vi "Control - Industrial Control.vi"() -> ()   [LabVIEW 2013, in "PID Control Workspace Object.lvlib"]
doc: "Sample numeric display item."
uses:
  Control Workspace Object Support.llb/PID Control Workspace Object.lvlib
  NationalInstruments.VeriStand.SystemStorage
  NationalInstruments.VeriStand.ClientAPI
  Control Workspace Object Support.llb/Constants.vi
  Control Workspace Object Support.llb/Control Addon Shared.lvlib
  Control Workspace Object Support.llb/NI_VS Workspace ExecutionAPI.lvlib
panel:
  in  "Manual State":bool
  in  "Manual Control":bool
  in  "Setpoint":dbl
  in  "NIVS.System Definition Root":refnum<k24>
  in  "NIVS.Gateway IP Address":string
  in  "Hold":bool
  in  "Autoscale Y":bool=TRUE
  in  "Autoscale X":bool=TRUE
  out "Chart":waveform(dbl)[](graph)
  out "Control Name":string
  in  "Item.Data":T1
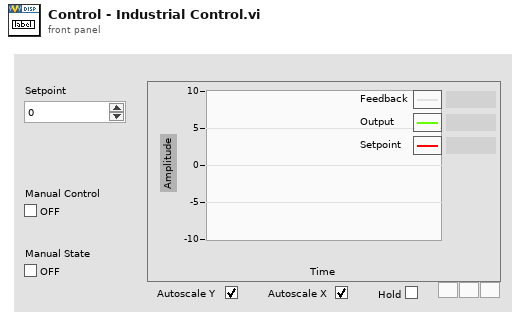
[diagram p1: front panel]
types:
  T1 = cluster{"Template VI":string, "Position X":i32, "Position Y":i32, "Custom":string, "Show Title Bar":bool, "ID":i32, "Always On Top":bool, "Allow Resize":bool, "Allow Minimize":bool, "Allow Close":bool, "Size to Screen":bool, "Screen.ID":i32, "State":enum16{"Normal", "New"}, "Title":string, "Window Bounds":cluster{"[0]":i16, "[1]":i16, "[2]":i16, "[3]":i16}, "Channel Ref":u64, "Unit":string, "Default Units?":bool, "Flash Limit?":bool, "Color 1":u32, "Color 2":u32, "Color 3":u32, "Color 4":u32, "Bck Color":u32, "Fore Color":u32, "Limit 1":dbl, "Limit 2":dbl, "Limit 3":dbl, "Limit 4":dbl, "Limit Mode 1":i32, "Limit Mode 2":i32, "Limit Mode 3":i32, "Limit Mode 4":i32, "Scale Precision":i32, "Scale Min":dbl, "Scale Max":dbl, "Format":i32, "Precision":i32, "Background Type":i32, "IDs":i32[], "Units":string[], "Labels":string[], "Scale Factor":dbl, "Scale Offset":dbl, "YScale Index":u32[], "XScale":cluster{"Format":u8, "Precision":u8, "Fit":u8, "Label":string, "Use Default Label":bool, "Label Visible":bool, "Min":dbl, "Max":dbl}, "YScales":cluster{"Format":u8, "Precision":u8, "Fit":u8, "Label":string, "Use Default Label":bool, "Label Visible":bool, "Min":dbl, "Max":dbl}[], "Plots":cluster{"Bar Style":u8, "Fill To":i16, "Fill/PtColor":u32, "Line Style":u8, "Line Width":u8, "Color":u32, "Interp":u8, "Point Style":u8}[], "Update Period":dbl, "History Length":dbl, "My.Ref":refnum<vi>, "Is Control?":bool, "Channel Paths":string[], "Custom Data":variant}
  T2 = enum8{"Idle", "Start Acq", "Run", "Stop Acq", "Exit"}
  T3 = cluster{"Action":enum8{"Idle", "Start Acq", "Run", "Stop Acq", "Exit"}, "Channels":string[]}
  T4 = cluster{"Initialized Waveform":waveform(dbl)[], "VS UDP Session":refnum<k24>, "Channel IDs":i32[], "Packet IDs":i32[], "Max Packet Size":i32, "UDP Ref":refnum<k16>}
  T5 = cluster{"Cached":cluster{"Path":string}, "Found?":bool, "UDP Channels":string[], "Connected?":bool, "Previous Values":dbl[], "Slow Channels":string[]}
  T6 = cluster{"Operation":enum16{"SetCustomData", "DeleteItem"}, "Data":variant}
  T7 = cluster{"CustDatRef":refnum<user-event>, "EvtRef":refnum<k27>}
  T8 = cluster{"Event Registration Refnum":refnum<event-registration>, "SystemChangeEventRef":refnum<event-registration>}
  T9 = cluster{"ID":i32, "t0":dbl, "dt":dbl, "Channel IDs":i32[], "Channel Data":dbl[][], "Sample Offset":u64}
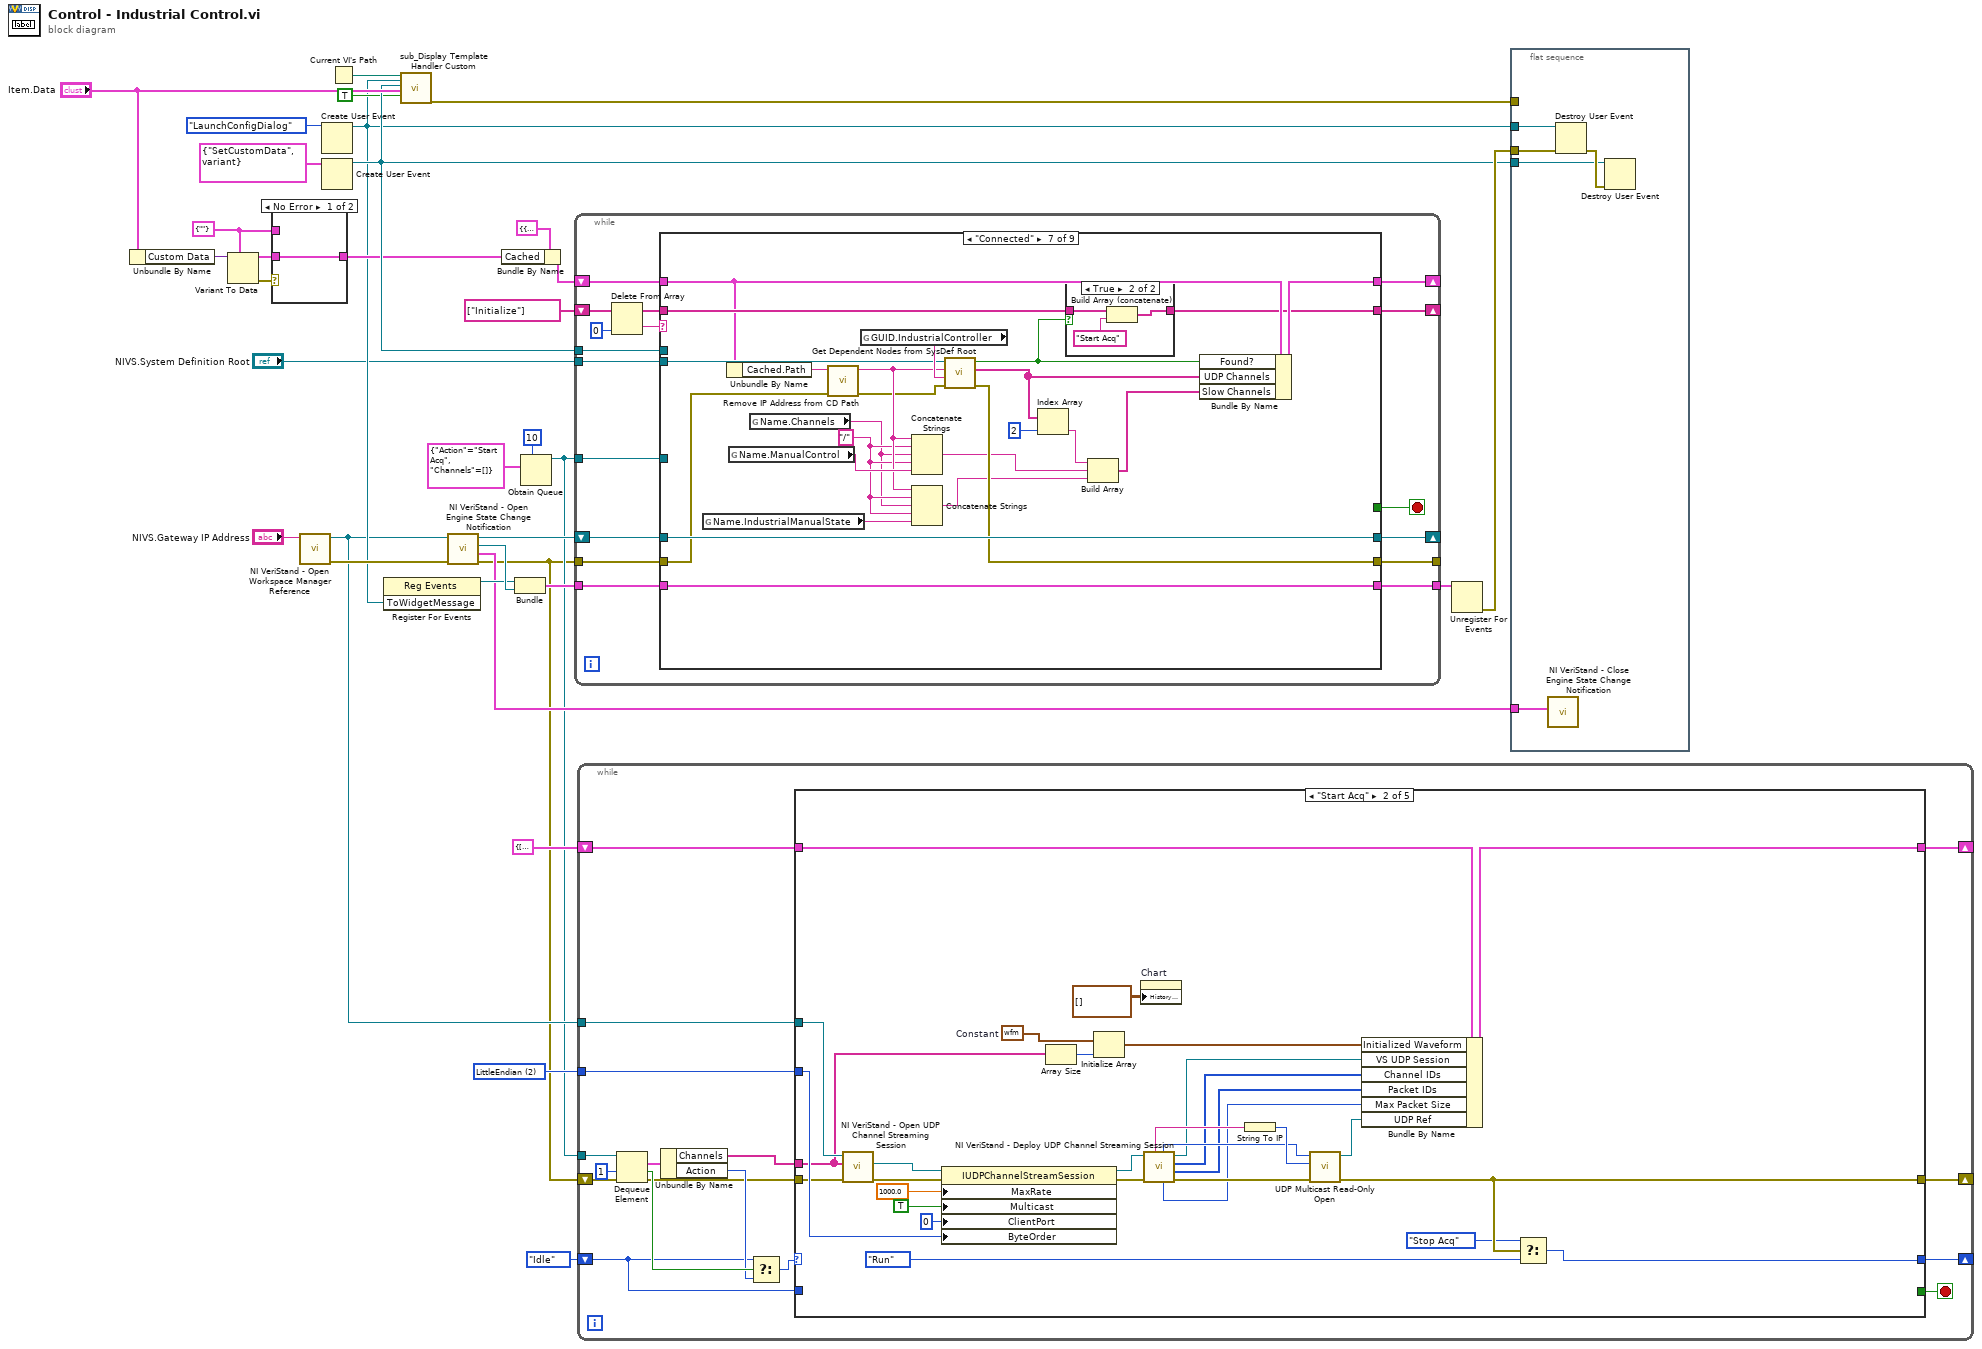
[diagram p0: block diagram]
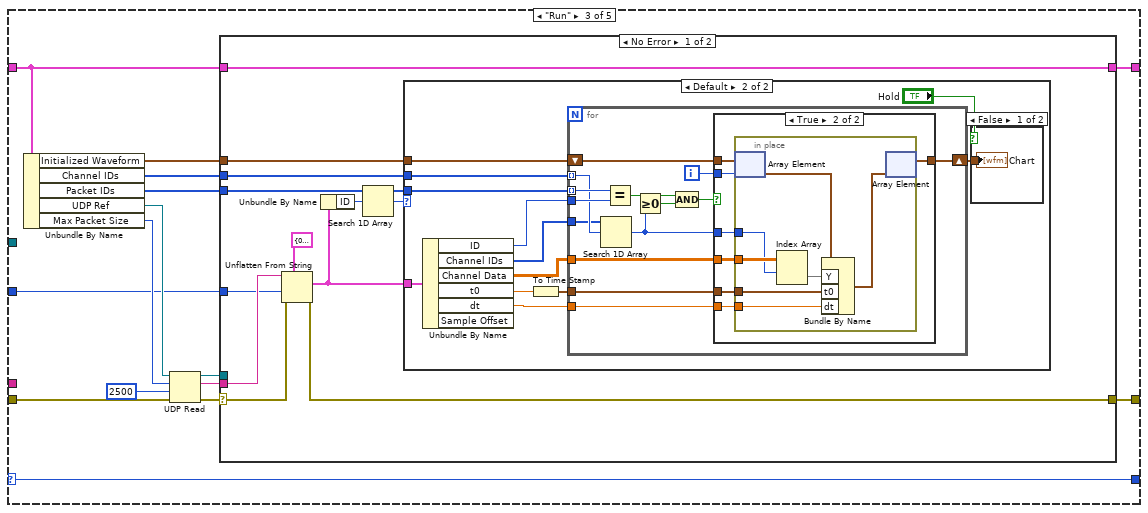
[diagram p3: hidden frame]
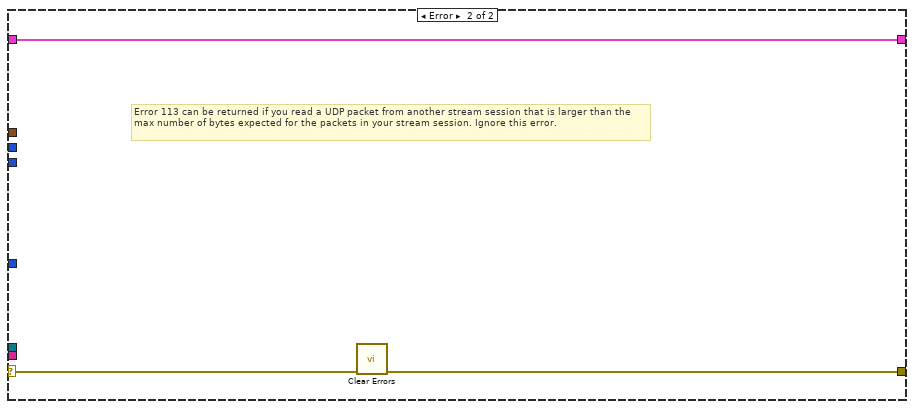
[diagram p7: hidden frame]
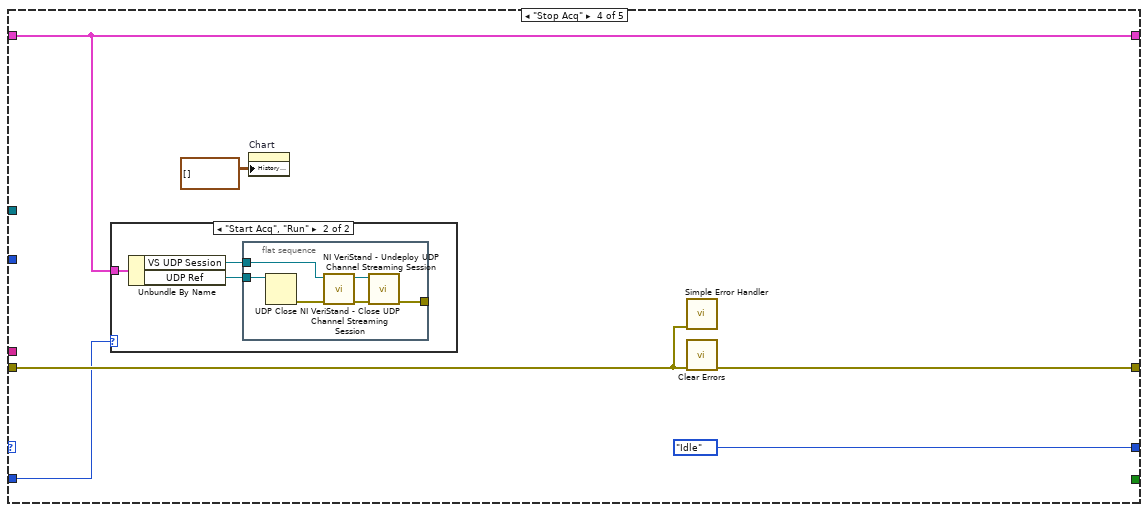
[diagram p8: hidden frame]
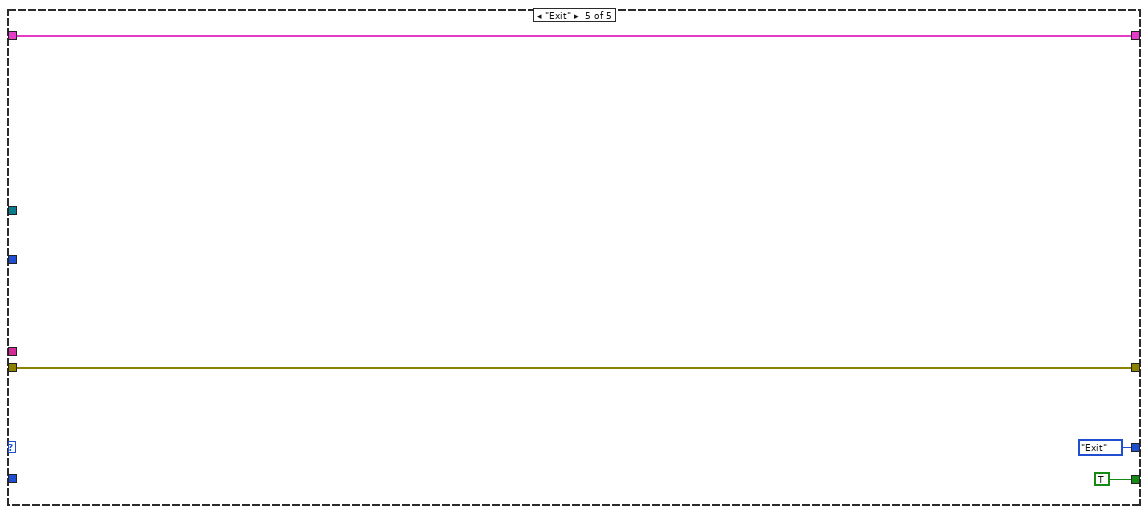
[diagram p10: hidden frame]
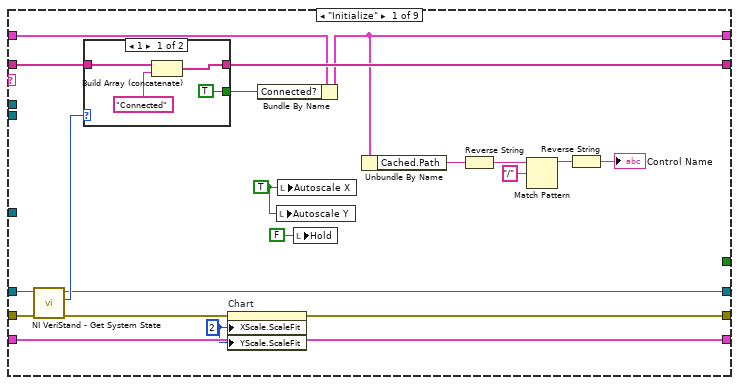
[diagram p12: hidden frame]
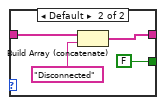
[diagram p13: hidden frame]
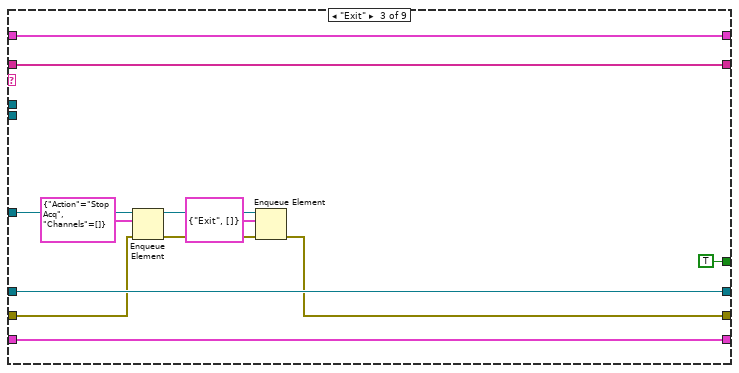
[diagram p15: hidden frame]
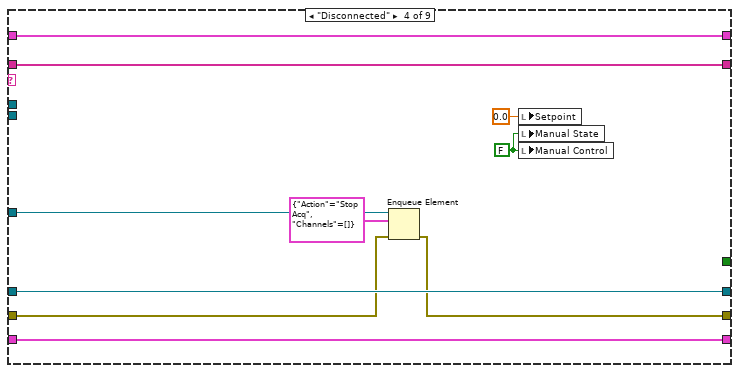
[diagram p16: hidden frame]
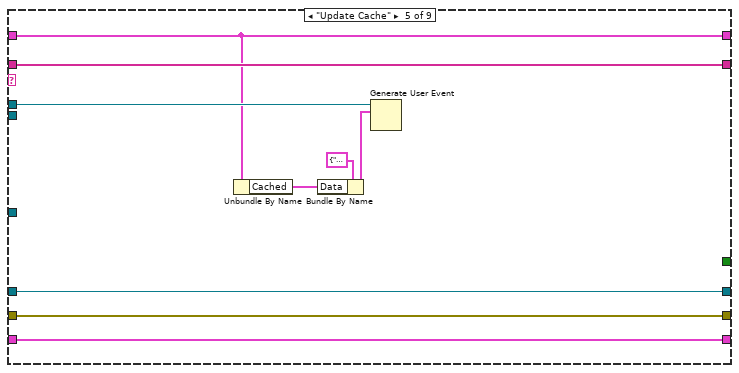
[diagram p17: hidden frame]
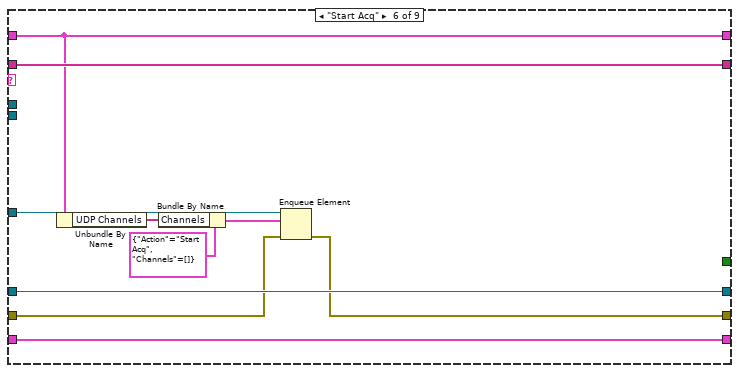
[diagram p18: hidden frame]
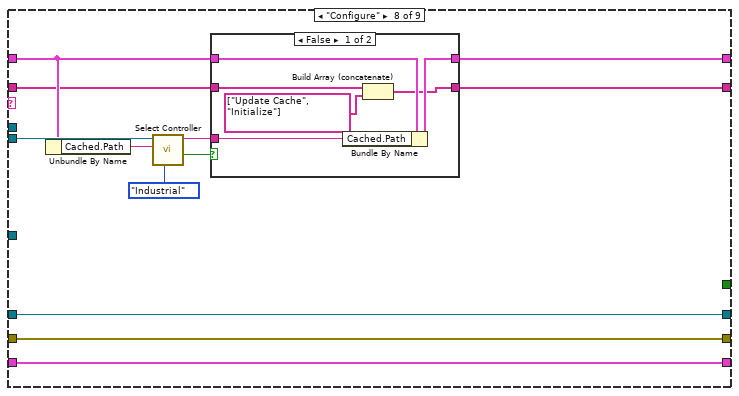
[diagram p20: hidden frame]
diagram:
  w6 = 2 items=["BigEndian", "NativeHostOrder", "LittleEndian"] ("Byte Order")
  w14 = cluster{"Path":string} {"Path"=""}
  n1 = Unbundle By Name("Item.Data") -> ("Custom Data"=w18:variant)
  n2 = Variant To Data(type=w14, Variant=w18) -> (data=w15:cluster{"Path":string}, error out=w16:errorcluster)  [unwired: 1 in]
  n3 = case shown="No Error" w16 {
    tunnel: w15 -> [w35 _]
    tunnel: [w35 w36] -> w11
    tunnel: w14 -> [_ w36]
    frame No Error {
    }
    frame Error {
    }
  }
  n4 = call "NI VeriStand - Open Workspace Manager Reference.vi"("Gateway IP Address (\"\": localhost)"="NIVS.Gateway IP Address") -> ("error out"=w25:errorcluster, "WorkspaceManager"=w8:refnum<k24>)  [unwired: 9 in]
  n5 = Create User Event(user event datatype=enum16{"Stop", "LaunchConfigDialog"}."LaunchConfigDialog" ("ToWidgetMessage")) -> (user event=w10:refnum<user-event>)  [unwired: 1 in, 1 out]
  n6 = Create User Event(user event datatype=T6 {"Operation"=enum."SetCustomData", "Data"=variant} ("Data")) -> (user event=w28:refnum<user-event>)  [unwired: 1 in, 1 out]
  n7 = Current VI's Path() -> (path=w30:path)
  n8 = register-events(w10) -> (reference out=w23:refnum<event-registration>)  [unwired: 2 in, 1 out]
  n9 = call "sub_Display Template Handler Custom.vi"("Parent.Path"=w30, "ToWidgetEvent"=w10, "ToWorkspace"=w28, "Item.Data"="Item.Data", "Resizable"=TRUE) -> ("error out"=w34:errorcluster)  [unwired: 14 in]
  n10 = call "NI VeriStand - Open Engine State Change Notification.vi"("error in (no error)"=w25, "WorkspaceManager in"=w8) -> ("error out"=w1:errorcluster, "SystemStateRefs"=w21:T7, "SystemChangeEventRef"=w24:refnum<event-registration>, "WorkspaceManager out"=w19:refnum<k24>)  [unwired: 6 in]
  n11 = Bundle By Name(cluster=T5 {"Cached"={"Path"=""}, "Found?"=FALSE, "UDP Channels"=[], "Connected?"=FALSE, "Previous Values"=[0.0, 0.0, 0.0], "Slow Channels"=[]}, "Cached"=w11) -> (w12:T5)
  n12 = Bundle("Event Registration Refnum"=w23, "SystemChangeEventRef"=w24) -> (w22:T8)  [unwired: 1 in]
  n13 = Obtain Queue(max queue size (-1, unlimited)=10, element data type=T3 {"Action"=enum."Start Acq", "Channels"=[]}) -> (queue out=w3:refnum<queue>)  [unwired: 3 in, 2 out]
  n14 = while {
    tunnel: w22 -> [w53]
    tunnel: w28 -> [w51]
    shift-right: [w45] -> _
    shift-left: string[] ["Initialize"] -> [w49]
    shift-right: [w43] -> _
    shift-left: w19 -> [w42]
    tunnel: w1 -> [w47]
    tunnel: [w44] -> w17
    tunnel: [w40] -> _
    shift-right: [w39] -> _
    shift-left: w12 -> [w41]
    tunnel: "NIVS.System Definition Root" -> [w38]
    tunnel: w3 -> [w37]
    stop <- w52 stop-if-true
    n15 = Delete From Array(array=w49, index=0) -> (deleted portion=w48:string, array with subset deleted=w46:string[])  [unwired: 1 in]
    n16 = case shown="\"Connected\"" w48 {
      tunnel: w53 -> [w67 w85 w97 w107 w116 w126 w150 w167 w186]
      tunnel: [_ _ TRUE _ _ _ _ _ _] -> w52
      tunnel: [w69 w86 w98 w108 w117 w127 w133 w157 w183] -> w45
      tunnel: w51 -> [_ _ _ _ w113 _ _ _ _]
      tunnel: w47 -> [w72 w83 w89 w103 w114 w119 w137 w165 w179]
      tunnel: w46 -> [w70 w86 w98 w108 w117 w127 w151 w156 w182]
      tunnel: [w67 w85 w97 w107 w116 w126 w150 w167 w184] -> w44
      tunnel: [w68 w84 w96 w106 w115 w125 w149 w166 w180] -> w43
      tunnel: w42 -> [w71 w84 w96 w106 w115 w125 w149 w166 w181]
      tunnel: w41 -> [w61 w82 w95 w105 w110 w124 w145 w161 w176]
      tunnel: [w55 w83 w88 w102 w114 w118 w148 w165 w178] -> w40
      tunnel: [w60 w82 w95 w105 w110 w124 w144 w160 w177] -> w39
      tunnel: w38 -> [_ _ _ _ _ _ w146 w163 _]
      tunnel: w37 -> [_ _ w94 w104 _ w123 _ _ _]
      frame "Initialize" {
        w57 = u8 2 ("X Scale.Scale Fit")
        w58 = TRUE ("Autoscale X")
        n17 = call "NI VeriStand - Get System State.vi"("error in (no error)"=w72, "WorkspaceManager in"=w71) -> ("error out"=w56:errorcluster, "System State"=w73:u8, "WorkspaceManager  out"=w68:refnum<k24>)  [unwired: 5 in, 2 out]
        n18 = case shown="1" w73 {
          tunnel: w70 -> [w77 w81]
          tunnel: [w76 w80] -> w69
          tunnel: [TRUE FALSE] -> w59
          frame 1 {
            n19 = Build Array (concatenate)(w77, "Connected") -> (w76:string[])
          }
          frame Default {
            n20 = Build Array (concatenate)(w81, "Disconnected") -> (w80:string[])
          }
        }
        n21 = property on="Chart" class="WFChart (strict)"(error in=w56, "XScale.ScaleFit"=w57, "YScale.ScaleFit"=w57) -> (error out=w55:errorcluster)  [unwired: 1 in, 1 out]
        n22 = Bundle By Name(cluster=w61, "Connected?"=w59) -> (w60:T5)
        n23 = local write "Autoscale Y"(w58) -> ()
        n24 = local write "Autoscale X"(w58) -> ()
        n25 = local write "Hold"(FALSE ("Hold")) -> ()
        n26 = Unbundle By Name(w60) -> ("Cached.Path"=w63:string)
        n27 = Reverse String(1:w63) -> (0:w66:string)
        n28 = Match Pattern(string=w66, regular expression="/") -> (before substring=w62:string)  [unwired: 1 in, 3 out]
        n29 = Reverse String(1:w62) -> (0:→"Control Name":string)
      }
      frame Default {
      }
      frame "Exit" {
        n30 = Enqueue Element(queue=w94, element=T3 {"Action"=enum."Stop Acq", "Channels"=[]}, error in (no error)=w89) -> (queue out=w92:refnum<queue>, error out=w90:errorcluster)  [unwired: 1 in, 1 out]
        n31 = Enqueue Element(queue=w92, element=T3 {"Action"=enum."Exit", "Channels"=[]}, error in (no error)=w90) -> (error out=w88:errorcluster)  [unwired: 1 in, 2 out]
      }
      frame "Disconnected" {
        w99 = FALSE ("Manual Control")
        n32 = Enqueue Element(queue=w104, element=T3 {"Action"=enum."Stop Acq", "Channels"=[]}, error in (no error)=w103) -> (error out=w102:errorcluster)  [unwired: 1 in, 2 out]
        n33 = local write "Setpoint"(0.0 ("Setpoint")) -> ()
        n34 = local write "Manual State"(w99) -> ()
        n35 = local write "Manual Control"(w99) -> ()
      }
      frame "Update Cache" {
        n36 = Unbundle By Name(w110) -> ("Cached"=w109:cluster{"Path":string})
        n37 = Bundle By Name(cluster=T6 {"Operation"=enum."SetCustomData", "Data"=variant} ("event data"), "Data"=w109) -> (w111:T6)
        n38 = Generate User Event(user event=w113, event data cluster=w111) -> ()  [unwired: 2 in, 2 out]
      }
      frame "Start Acq" {
        n39 = Unbundle By Name(w124) -> ("UDP Channels"=w121:string[])
        n40 = Bundle By Name(cluster=T3 {"Action"=enum."Start Acq", "Channels"=[]}, "Channels"=w121) -> (w120:T3)
        n41 = Enqueue Element(queue=w123, element=w120, error in (no error)=w119) -> (error out=w118:errorcluster)  [unwired: 1 in, 2 out]
      }
      frame "Connected" {
        w130 = "/" ("string")
        n42 = global read "Constants.vi" "Name.IndustrialManualState"() -> (w140:string)
        n43 = Unbundle By Name(w145) -> ("Cached.Path"=w143:string)
        n44 = global read "Constants.vi" "Name.ManualControl"() -> (w142:string)
        n45 = global read "Constants.vi" "Name.Channels"() -> (w129:string)
        n46 = call "Remove IP Address from CD Path.vi"("error in (no error)"=w137, "CD Path"=w143) -> ("error out"=w136:errorcluster, "Path"=w141:string)  [unwired: 8 in]
        n47 = global read "Constants.vi" "GUID.IndustrialController"() -> (w147:string)
        n48 = Concatenate Strings(w141, w130, w129, w130, w142) -> (w139:string)
        n49 = Concatenate Strings(w141, w130, w129, w130, w140) -> (w138:string)
        n50 = call "Get Dependent Nodes from SysDef Root.vi"("error in (no error)"=w136, "GUID"=w147, "Path"=w141, "SysDef Ref"=w146) -> ("error out"=w148:errorcluster, "Channels"=w132:string[], "Found"=w128:bool)  [unwired: 5 in]
        n51 = Index Array(array=w132, index=2) -> (element=w134:string)
        n52 = case shown="True" w128 {
          tunnel: w151 -> [w152 w155]
          tunnel: [w152 w154] -> w133
          frame False {
          }
          frame True {
            n53 = Build Array (concatenate)(w155, "Start Acq") -> (w154:string[])
          }
        }
        n54 = Build Array(w134, w139, w138) -> (w131:string[])
        n55 = Bundle By Name(cluster=w145, "Found?"=w128, "UDP Channels"=w132, "Slow Channels"=w131) -> (w144:T5)
      }
      frame "Configure" {
        n56 = Unbundle By Name(w161) -> ("Cached.Path"=w162:string)
        n57 = call "Select Controller.vi"("Type"=enum16{"PID", "Industrial"}."Industrial", "CD Path"=w162, "NIVS.System Definition Root"=w163) -> ("Cancelled?"=w159:bool, "Custom Device Path Out"=w158:string)  [unwired: 6 in, 1 out]
        n58 = case shown="False" w159 {
          tunnel: w161 -> [w173 w174]
          tunnel: [w172 w174] -> w160
          tunnel: w158 -> [w171 _]
          tunnel: [w169 w175] -> w157
          tunnel: w156 -> [w170 w175]
          frame False {
            n59 = Bundle By Name(cluster=w173, "Cached.Path"=w171) -> (w172:T5)
            n60 = Build Array (concatenate)(w170, string[] ["Update Cache", "Initialize"]) -> (w169:string[])
          }
          frame True {
          }
        }
      }
      frame "" {
        n61 = event shown="[2] \"Setpoint\", \"Manual Control\", \"Manual State\": Value Change" {
          selector: w186 -> [_ _ _ _ _]
          dyn-events: [_ _ _ _ _] -> w184
          timeout: 100 -> [_ _ _ _ _]
          tunnel: [w205 w227 w245 w274 w294] -> w183
          tunnel: w182 -> [w205 w227 w245 w275 w293]
          tunnel: w181 -> [w202 w226 w238 w278 w295]
          tunnel: [w201 w226 w237 w277 w295] -> w180
          tunnel: w179 -> [w204 w220 w240 w280 w292]
          tunnel: [w203 w219 w239 w279 w292] -> w178
          tunnel: [w198 w225 w233 w272 w291] -> w177
          tunnel: w176 -> [w199 w225 w233 w273 w291]
          event Timeout {
            n62 = event-data() -> ()  [unwired: 2 out]
            n63 = Unbundle By Name(w199) -> ("Found?"=w191:bool, "Connected?"=w197:bool, "Slow Channels"=w200:string[])
            n64 = Compound Arithmetic op=AND(w191, w197) -> (w192:bool)
            n65 = case shown="True" w192 {
              tunnel: w204 -> [w208 w214]
              tunnel: [w208 w213] -> w203
              tunnel: w202 -> [w207 w212]
              tunnel: [w207 w211] -> w201
              tunnel: w200 -> [_ w210]
              tunnel: [dbl[] [0.0, 0.0, 0.0] ("Values") w209] -> w196
              frame False {
              }
              frame True {
                n66 = call "NI VeriStand - Get Multiple Channel Values.vi"("error in (no error)"=w214, "Channels"=w210, "WorkspaceManager in"=w212) -> ("error out"=w213:errorcluster, "Values"=w209:dbl[], "WorkspaceManager out"=w211:refnum<k24>)  [unwired: 6 in]
              }
            }
            n67 = Index Array(array=w196) -> (element #1=w195:dbl, element #2=w190:dbl, element #3=w189:dbl)  [unwired: 3 in]
            n68 = To Long Integer(number=w190) -> (32bit integer=w194:i32)
            n69 = To Long Integer(number=w189) -> (32bit integer=w187:i32)
            n70 = Not Equal To 0?(x=w194) -> (x != 0?=w193:bool)
            n71 = Not Equal To 0?(x=w187) -> (x != 0?=w188:bool)
            n72 = local write "Setpoint"(w195) -> ()
            n73 = local write "Manual Control"(w193) -> ()
            n74 = local write "Manual State"(w188) -> ()
            n75 = Bundle By Name(cluster=w199, "Previous Values"=w196) -> (w198:T5)
          }
          event "Autoscale Y", "Autoscale X": Value Change {
            n76 = event-data() -> ()  [unwired: 2 out]
            n77 = Select(t=u8 2, s="Autoscale X", f=u8 0 ("X Scale.Scale Fit")) -> (s? t:f=w222:u8)
            n78 = Select(t=u8 2, s="Autoscale Y", f=u8 0 ("X Scale.Scale Fit")) -> (s? t:f=w215:u8)
            n79 = property on="Chart" class="WFChart (strict)"(error in=w220, "XScale.ScaleFit"=w222, "YScale.ScaleFit"=w215) -> (error out=w219:errorcluster)  [unwired: 1 in, 1 out]
          }
          event "Setpoint", "Manual Control", "Manual State": Value Change {
            n80 = event-data() -> ()  [unwired: 2 out]
            n81 = Unbundle By Name(w233) -> ("Found?"=w231:bool, "Connected?"=w235:bool, "Previous Values"=w234:dbl[], "Slow Channels"=w236:string[])
            n82 = Boolean To (0,1)(Boolean="Manual Control") -> (0, 1=w230:i16)
            n83 = Boolean To (0,1)(Boolean="Manual State") -> (0, 1=w228:i16)
            n84 = Build Array("Setpoint", w230, w228) -> (w241:dbl[])
            n85 = Not Equal?(x=w234, y=w241) -> (x != y?=w244:bool[])
            n86 = Compound Arithmetic op=AND(w231, w235) -> (w232:bool)
            n87 = case shown="True" w232 {
              tunnel: w244 -> [_ w254]
              tunnel: w241 -> [_ w253]
              tunnel: w240 -> [w247 w252]
              tunnel: [w247 w251] -> w239
              tunnel: w238 -> [w246 w250]
              tunnel: [w246 w249] -> w237
              tunnel: w236 -> [_ w248]
              frame False {
              }
              frame True {
                n88 = for {
                  shift-right: [w260] -> w251
                  shift-left: w252 -> [w261]
                  shift-right: [w259] -> w249
                  shift-left: w250 -> [w258]
                  tunnel: w254 -> [w257] mode=indexing
                  tunnel: w253 -> [w256] mode=indexing
                  tunnel: w248 -> [w255] mode=indexing
                  n89 = case shown="False" w257 {
                    tunnel: w261 -> [w263 w269]
                    tunnel: [w263 w268] -> w260
                    tunnel: [w262 w267] -> w259
                    tunnel: w258 -> [w262 w266]
                    tunnel: w256 -> [_ w265]
                    tunnel: w255 -> [_ w264]
                    frame False {
                    }
                    frame True {
                      n90 = call "NI VeriStand - Set Single Channel Value.vi"("error in (no error)"=w269, "Value"=w265, "Channel"=w264, "WorkspaceManager in"=w266) -> ("error out"=w268:errorcluster, "WorkspaceManager out"=w267:refnum<k24>)  [unwired: 6 in]
                    }
                  }
                }
              }
            }
          }
          event User Event {
            n91 = event-data() -> ()  [unwired: 2 out]
            n92 = call "NI VeriStand - Get System State.vi"("error in (no error)"=w280, "WorkspaceManager in"=w278) -> ("error out"=w279:errorcluster, "System State"=w276:u8, "WorkspaceManager  out"=w277:refnum<k24>)  [unwired: 5 in, 2 out]
            n93 = case shown="Default" w276 {
              tunnel: w275 -> [w285 w290]
              tunnel: [w284 w289] -> w274
              tunnel: [w282 w287] -> w271
              tunnel: w273 -> [w282 w287]
              tunnel: [TRUE FALSE] -> w270
              frame 1 {
                n94 = Build Array (concatenate)(w285, "Connected") -> (w284:string[])
              }
              frame Default {
                n95 = Build Array (concatenate)(w290, "Disconnected") -> (w289:string[])
              }
            }
            n96 = Bundle By Name(cluster=w271, "Connected?"=w270) -> (w272:T5)
          }
          event User Event {
            n97 = event-data() -> ("ToWidgetMessage"=w296:enum16{"Stop", "LaunchConfigDialog"})  [unwired: 1 out]
            n98 = case shown="\"Stop\"" w296 {
              tunnel: [w297 w299 w302] -> w294
              tunnel: w293 -> [w297 w300 w303]
              frame Default {
              }
              frame "Stop" {
                n99 = Build Array (concatenate)(w300, "Exit") -> (w299:string[])
              }
              frame "LaunchConfigDialog" {
                n100 = Build Array (concatenate)(w303, "Configure") -> (w302:string[])
              }
            }
          }
        }
      }
    }
  }
  n101 = while {
    tunnel: w8 -> [w320]
    tunnel: w6 -> [w318]
    tunnel: w3 -> [w317]
    shift-right: [w311] -> _
    shift-left: T2."Idle" ("Action") -> [w304]
    shift-right: [w310] -> _
    shift-left: T4 {"Initialized Waveform"=[], "VS UDP Session"=refnum, "Channel IDs"=[], "Packet IDs"=[], "Max Packet Size"=0, "UDP Ref"=refnum} -> [w319]
    shift-right: [w307] -> _
    shift-left: w1 -> [w306]
    stop <- w309 stop-if-true
    n102 = Dequeue Element(queue=w317, timeout in ms (-1)=1, error in (no error)=w306) -> (element=w316:T3, timed out?=w314:bool, error out=w308:errorcluster)  [unwired: 1 out]
    n103 = Unbundle By Name(w316) -> ("Channels"=w305:string[], "Action"=w313:T2)
    n104 = Select(t=w304, s=w314, f=w313) -> (s? t:f=w312:T2)
    n105 = case shown="\"Start Acq\"" w312 {
      selector: w312 -> [w321 _ w357 _ _]
      tunnel: w320 -> [_ w341 _ _ _]
      tunnel: w319 -> [w323 w340 w358 w431 w442]
      tunnel: w318 -> [_ w333 w354 _ _]
      tunnel: [w323 w332 w359 w431 w442] -> w310
      tunnel: [w321 w327 w357 T2."Idle" ("Action") T2."Exit" ("Action")] -> w311
      tunnel: [_ _ _ _ TRUE] -> w309
      tunnel: w308 -> [w322 w331 w356 w429 w441]
      tunnel: [w322 w330 w355 w428 w441] -> w307
      tunnel: w305 -> [_ w325 _ _ _]
      tunnel: w304 -> [_ _ _ w427 _]
      frame "Idle" {
      }
      frame "Start Acq" {
        w347 = waveform(dbl) {"t0"=timestamp(0 s since 1904-01-01), "dt"=1.0, "Y"=[]}  # Constant
        n106 = call "NI VeriStand - Open UDP Channel Streaming Session.vi"("error in (no error)"=w331, "Channels"=w325, "WorkspaceManager in"=w341) -> ("error out"=w351:errorcluster, "UDPChannelStreamSession out"=w348:refnum<k24>)  [unwired: 6 in, 1 out]
        n107 = property class="IUDPChannelStreamSession"(reference=w348, error in=w351, "MaxRate"=1000.0, "Multicast"=TRUE, "ClientPort"=u16 0, "ByteOrder"=w333) -> (reference out=w350:refnum<k24>, error out=w349:errorcluster)
        n108 = Array Size(array=w325) -> (size(s)=w346:i32)
        n109 = Initialize Array(w347, w346) -> (w339:waveform(dbl)[])
        n110 = property on="Chart" class="WFChart (strict)"("History Data"=waveform(dbl)[][] []) -> ()  [unwired: 2 in, 2 out]
        n111 = call "NI VeriStand - Deploy UDP Channel Streaming Session.vi"("error in (no error)"=w349, "UDPChannelStreamSession in"=w350) -> ("error out"=w343:errorcluster, "Packet IDs"=w336:i32[], "Channel IDs"=w337:i32[], "UDPChannelStreamSession out"=w338:refnum<k24>, "Max Packet Size"=w335:i32, "Port"=w344:u16, "UDP Multicast Address"=w342:string)  [unwired: 3 in]
        n112 = String To IP(1:w342) -> (0:w345:u32)
        n113 = call "UDP Multicast Read-Only Open.vi"("error in (no error)"=w343, "multicast addr"=w345, "port"=w344) -> ("error out"=w330:errorcluster, "connection ID"=w334:refnum<k16>)  [unwired: 6 in, 1 out]
        n114 = Bundle By Name(cluster=w340, "Initialized Waveform"=w339, "VS UDP Session"=w338, "Channel IDs"=w337, "Packet IDs"=w336, "Max Packet Size"=w335, "UDP Ref"=w334) -> (w332:T4)
        n115 = Select(t=T2."Stop Acq", s=w330, f=T2."Run" ("Action")) -> (s? t:f=w327:T2)
      }
      frame "Run" {
        n116 = Unbundle By Name(w358) -> ("Initialized Waveform"=w364:waveform(dbl)[], "Channel IDs"=w363:i32[], "Packet IDs"=w362:i32[], "UDP Ref"=w361:refnum<k16>, "Max Packet Size"=w360:i32)
        n117 = UDP Read(connection ID=w361, max size (548)=w360, timeout ms (25000)=2500, 8:w356) -> (data out=w366:string, error out=w367:errorcluster, 3:w368:refnum<k16>)  [unwired: 2 out]
        n118 = case shown="No Error" w367 {
          selector: w367 -> [w379 w425]
          tunnel: w362 -> [w374 _]
          tunnel: w366 -> [w377 _]
          tunnel: w363 -> [w376 _]
          tunnel: w364 -> [w375 _]
          tunnel: [w380 w423] -> w355
          tunnel: w368 -> [_ _]
          tunnel: w354 -> [w370 _]
          tunnel: [w369 w424] -> w359
          tunnel: w358 -> [w369 w424]
          frame No Error {
            n119 = Unflatten From String(type=T9 {"ID"=0, "t0"=0.0, "dt"=0.0, "Channel IDs"=[], "Channel Data"=[], "Sample Offset"=0} ("UDP Data Packet"), binary string=w377, byte order (0:big-endian, network order)=w370, error in (no error)=w379) -> (value=w371:T9, error out=w380:errorcluster)  [unwired: 1 in, 1 out]
            n120 = Unbundle By Name(w371) -> ("ID"=w372:i32)
            n121 = Search 1D Array(1D array=w374, element=w372) -> (index of element=w373:i32)  [unwired: 1 in]
            n122 = case shown="Default" w373 {
              tunnel: w376 -> [_ w392]
              tunnel: w375 -> [_ w391]
              tunnel: w374 -> [_ w389]
              tunnel: w371 -> [_ w388]
              frame -1 {
                # "This is a packet from a different UDP session. Ignore it."
              }
              frame Default {
                n123 = Unbundle By Name(w388) -> ("ID"=w387:i32, "Channel IDs"=w386:i32[], "Channel Data"=w385:dbl[][], "t0"=w384:dbl, "dt"=w383:dbl)  [unwired: 1 out]
                n124 = To Time Stamp(1:w384) -> (0:w390:timestamp)
                n125 = for {
                  tunnel: w392 -> [w405] mode=indexing
                  tunnel: w389 -> [w407] mode=indexing
                  tunnel: w387 -> [w406]
                  tunnel: w385 -> [w399]
                  tunnel: w386 -> [w398]
                  shift-right: [w394] -> w382
                  shift-left: w391 -> [w397]
                  tunnel: w390 -> [w396]
                  tunnel: w383 -> [w395]
                  i -> [w400]
                  n126 = Search 1D Array(1D array=w398, element=w405) -> (index of element=w401:i32)  [unwired: 1 in]
                  n127 = Equal?(x=w407, y=w406) -> (x = y?=w404:bool)
                  n128 = Greater Or Equal To 0?(x=w401) -> (x >= 0?=w403:bool)
                  n129 = Compound Arithmetic op=AND(w404, w403) -> (w402:bool)
                  n130 = case shown="True" w402 {
                    tunnel: w401 -> [_ w413]
                    tunnel: w400 -> [_ w409]
                    tunnel: w399 -> [_ w414]
                    tunnel: w397 -> [w408 w415]
                    tunnel: w396 -> [_ w412]
                    tunnel: w395 -> [_ w411]
                    tunnel: [w408 w410] -> w394
                    frame False {
                      # "This channel is not in this UDP Data Packet."
                    }
                    frame True {
                      n131 = in-place {
                        in-place-border: w414 -> [w421]
                        in-place-border: w413 -> [w420]
                        in-place-border: w412 -> [w418]
                        in-place-border: w411 -> [w417]
                        n132 = in-place-array #1(w415, w409) -> (w422:waveform(dbl))
                        n133 = Index Array(array=w421, index (row)=w420) -> (element=w419:dbl[])  [unwired: 1 in]
                        n134 = Bundle By Name(cluster=w422, "Y"=w419, "t0"=w418, "dt"=w417) -> (w416:waveform(dbl))
                        n135 = in-place-array #1(w416) -> (w410:waveform(dbl)[])  [unwired: 1 out]
                      }
                    }
                  }
                }
                n136 = case shown="False" "Hold" {
                  tunnel: w382 -> [w393 _]
                  frame False {
                    "Chart" <- w393
                  }
                  frame True {
                  }
                }
              }
            }
          }
          frame Error {
            # "Error 113 can be returned if you read a UDP packet from another stream session that is larger than the max number of bytes expected for the packets in your stream session. Ignore this error."
            n137 = call "Clear Errors.vi"("error in (no error)"=w425) -> ("error out"=w423:errorcluster)  [unwired: 6 in]
          }
        }
      }
      frame "Stop Acq" {
        n138 = case shown="\"Start Acq\", \"Run\"" w427 {
          tunnel: w431 -> [_ w432]
          frame Default {
          }
          frame "Start Acq", "Run" {
            n139 = Unbundle By Name(w432) -> ("VS UDP Session"=w433:refnum<k24>, "UDP Ref"=w434:refnum<k16>)
            n140 = flat-sequence {
              tunnel: w434 -> [w437]
              tunnel: w433 -> [w436]
              tunnel: [w435] -> _
              frame #0 {
                n141 = UDP Close(connection ID=w437) -> (error out=w440:errorcluster)  [unwired: 1 in, 1 out]
                n142 = call "NI VeriStand - Undeploy UDP Channel Streaming Session.vi"("error in (no error)"=w440, "UDPChannelStreamSession in"=w436) -> ("error out"=w438:errorcluster, "UDPChannelStreamSession out"=w439:refnum<k24>)  [unwired: 8 in]
                n143 = call "NI VeriStand - Close UDP Channel Streaming Session.vi"("error in (no error)"=w438, "UDPChannelStreamSession in"=w439) -> ("error out"=w435:errorcluster)  [unwired: 9 in]
              }
            }
          }
        }
        n144 = property on="Chart" class="WFChart (strict)"("History Data"=waveform(dbl)[][] []) -> ()  [unwired: 2 in, 2 out]
        n145 = call "Simple Error Handler.vi"("error in (no error)"=w429) -> ()  [unwired: 4 in, 5 out]
        n146 = call "Clear Errors.vi"("error in (no error)"=w429) -> ("error out"=w428:errorcluster)  [unwired: 6 in]
      }
      frame "Exit" {
      }
    }
  }
  n147 = Unregister For Events(event registration refnum=w17) -> (error out=w32:errorcluster)  [unwired: 1 in]
  n148 = flat-sequence {
    tunnel: w34 -> [_]
    tunnel: w32 -> [w448]
    tunnel: w10 -> [w449]
    tunnel: w28 -> [w446]
    tunnel: w21 -> [w445]
    frame #0 {
      n149 = call "NI VeriStand - Close Engine State Change Notification.vi"("SystemStateRefs"=w445) -> ()  [unwired: 10 in, 1 out]
      n150 = Destroy User Event(user event=w449, error in=w448) -> (error out=w447:errorcluster)
      n151 = Destroy User Event(user event=w446, error in=w447) -> ()  [unwired: 1 out]
    }
  }
